vi "Intake Shooter Teleop.vi"(11 "Buttons":bool[](array[boolean])) -> ()   [LabVIEW 2019]
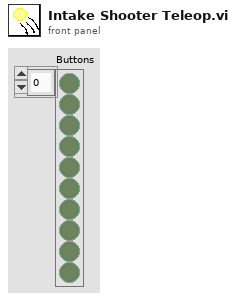
[diagram p1: front panel]
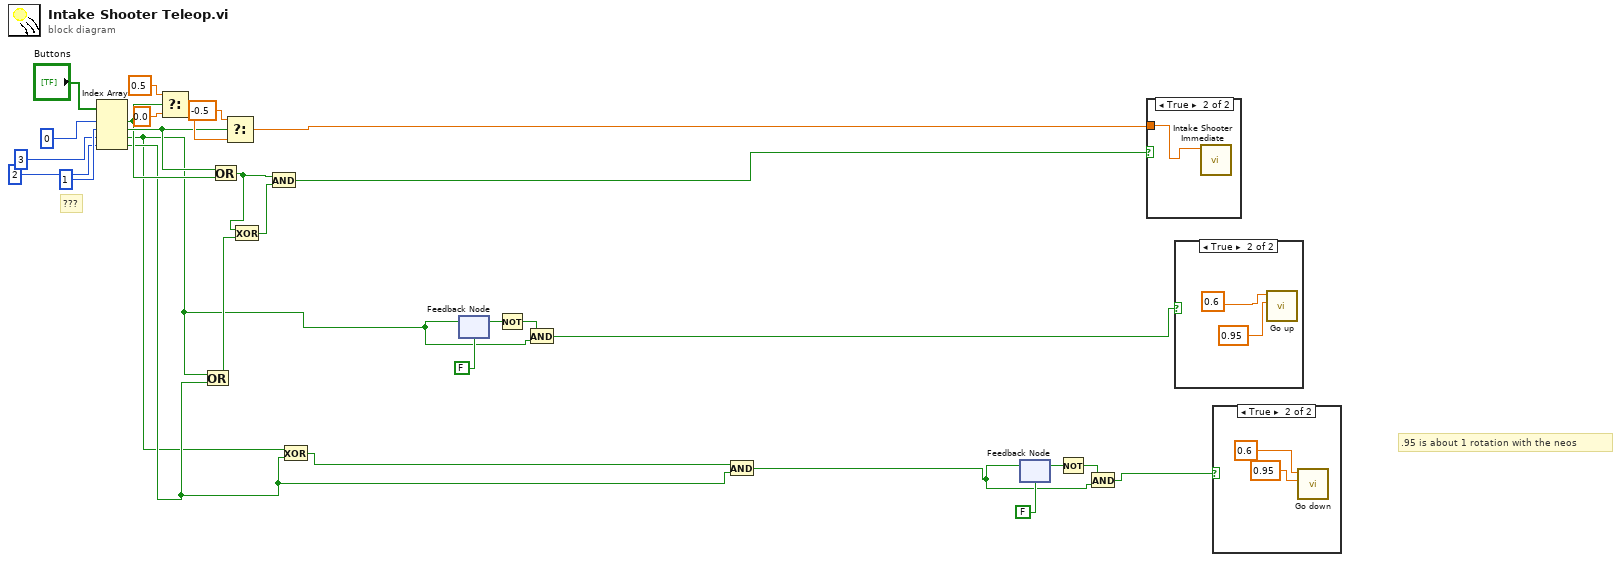
[diagram p0: block diagram]
diagram:
  # ".95 is about 1 rotation with the neos"
  # "???"
  n1 = Index Array(array="Buttons", index #1=0 ("index"), index #2=1 ("index"), index #3=3 ("index"), index #4=2 ("index")) -> (element #1=w20:bool, element #2=w21:bool, element #3=w2:bool, element #4=w11:bool)
  n2 = Select(t=0.5, s=w20, f=0.0) -> (s? t:f=w25:dbl)
  n3 = Or(x=w2, y=w11) -> (x .or. y?=w16:bool)
  n4 = Or(x=w21, y=w20) -> (x .or. y?=w14:bool)
  n5 = Select(t=-0.5, s=w21, f=w25) -> (s? t:f=w19:dbl)
  n6 = Exclusive Or(1:w16, 2:w14) -> (0:w15:bool)
  n7 = And(x=w14, y=w15) -> (x .and. y?=w13:bool)
  n8 = Exclusive Or(1:w11, 2:w2) -> (0:w12:bool)
  n9 = feedback #1(FALSE) -> (w9:bool)
  n10 = feedback-in #1(w2) -> ()
  n11 = Not(x=w9) -> (.not. x?=w10:bool)
  n12 = And(x=w10, y=w2) -> (x .and. y?=w1:bool)
  n13 = And(x=w12, y=w11) -> (x .and. y?=w4:bool)
  n14 = feedback #2(FALSE) -> (w6:bool)
  n15 = feedback-in #2(w4) -> ()
  n16 = Not(x=w6) -> (.not. x?=w7:bool)
  n17 = And(x=w7, y=w4) -> (x .and. y?=w3:bool)
  n18 = case shown="True" w13 {
    tunnel: w19 -> [_ w29]
    frame False {
    }
    frame True {
      n19 = call "Intake Shooter Immediate.vi"("Intake joystick"=w29) -> ()  [unwired: 10 in, 1 out]
    }
  }
  n20 = case shown="True" w1 {
    frame False {
    }
    frame True {
      n21 = call "Go up.vi"("Distance"=0.95, "Speed"=0.6 ("Setpoint")) -> ()  [unwired: 9 in, 1 out]
    }
  }
  n22 = case shown="True" w3 {
    frame False {
    }
    frame True {
      n23 = call "Go down.vi"("Distance"=0.95, "Speed"=0.6 ("Setpoint")) -> ()  [unwired: 9 in, 1 out]
    }
  }
